vi "Moving Window Waveform Smoother.vi"(9 "Points / Aperture(S)":dbl, 10 "Filter Mode":T1(ring), 11 "Raw Waveforms":waveform(dbl)[](array[waveform])) -> (3 "Filtered Waveforms":waveform(dbl)[](array[waveform]))   [LabVIEW 2010]
uses:
  <vilib>/Analysis/NI_AALBase.lvlib
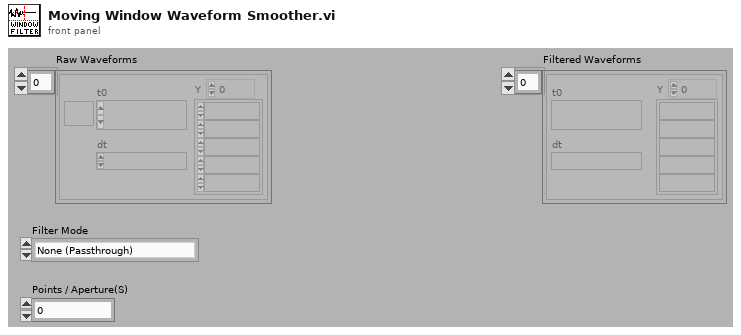
[diagram p1: front panel]
types:
  T1 = enum16{"None (Passthrough)", "Moving Window (Fixed)", "Moving Window (Time)"}
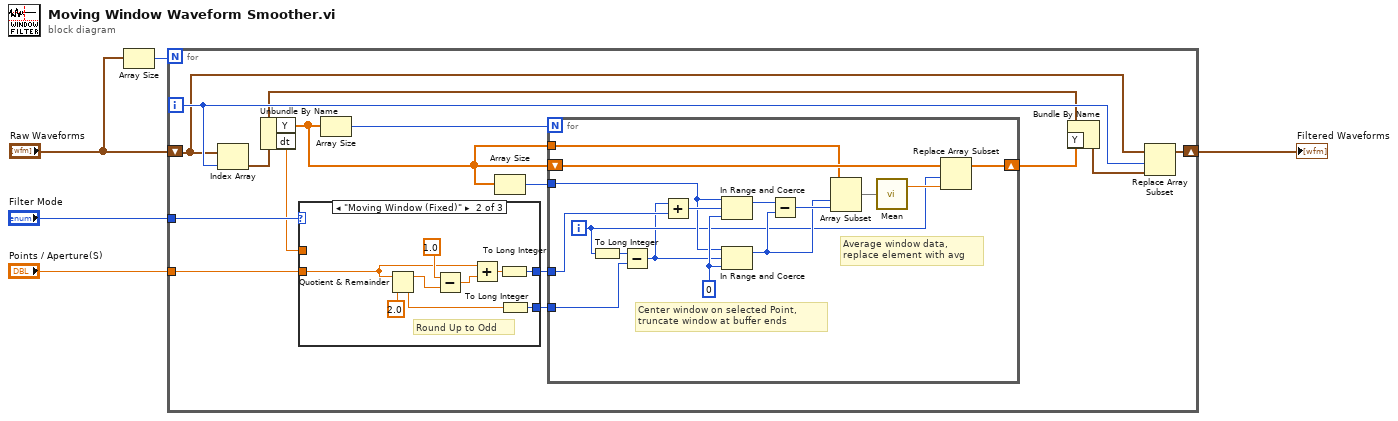
[diagram p0: block diagram]
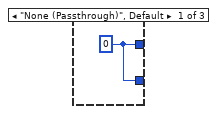
[diagram p2: hidden frame]
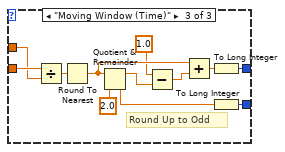
[diagram p3: hidden frame]
diagram:
  n1 = Array Size(array="Raw Waveforms") -> (size(s)=w4:i32)
  n2 = for {
    N: w4 -> [_]
    shift-right: [w9] -> w5
    shift-left: "Raw Waveforms" -> [w18]
    tunnel: "Filter Mode" -> [w13]
    tunnel: "Points / Aperture(S)" -> [w10]
    i -> [w19]
    n3 = Index Array(array=w18, index=w19) -> (element=w16:waveform(dbl))
    n4 = Unbundle By Name(w16) -> ("Y"=w8:dbl[], "dt"=w12:dbl)
    n5 = case shown="\"Moving Window (Fixed)\"" w13 {
      tunnel: w12 -> [_ _ w40]
      tunnel: [w20 w23 w38] -> w11
      tunnel: w10 -> [_ w24 w41]
      tunnel: [w20 w21 w31] -> w6
      frame "None (Passthrough)", Default {
        w20 = 0 ("Points / Aperture(uS)")
      }
      frame "Moving Window (Fixed)" {
        # "Round Up to Odd"
        n6 = Quotient & Remainder(x=w24, y=2.0) -> (x-y*floor(x/y)=w25:dbl, floor(x/y)=w22:dbl)
        n7 = Subtract(x=1.0 ("y"), y=w25) -> (x-y=w27:dbl)
        n8 = Add(x=w24, y=w27) -> (x+y=w28:dbl)
        n9 = To Long Integer(number=w28) -> (32bit integer=w23:i32)
        n10 = To Long Integer(number=w22) -> (32bit integer=w21:i32)
      }
      frame "Moving Window (Time)" {
        # "Round Up to Odd"
        n11 = Divide(x=w41, y=w40) -> (x/y=w39:dbl)
        n12 = Round To Nearest(number=w39) -> (nearest integer value=w36:dbl)
        n13 = Quotient & Remainder(x=w36, y=2.0) -> (x-y*floor(x/y)=w32:dbl, floor(x/y)=w30:dbl)
        n14 = Subtract(x=1.0 ("y"), y=w32) -> (x-y=w34:dbl)
        n15 = Add(x=w36, y=w34) -> (x+y=w35:dbl)
        n16 = To Long Integer(number=w35) -> (32bit integer=w38:i32)
        n17 = To Long Integer(number=w30) -> (32bit integer=w31:i32)
      }
    }
    n18 = Array Size(array=w8) -> (size(s)=w17:i32)
    n19 = Array Size(array=w8) -> (size(s)=w7:i32)
    n20 = for {
      N: w17 -> [_]
      shift-right: [w57] -> w14
      shift-left: w8 -> [w56]
      tunnel: w11 -> [w51]
      tunnel: w8 -> [w55]
      tunnel: w7 -> [w49]
      tunnel: w6 -> [w43]
      i -> [w45]
      w52 = 0 ("lower limit")
      # "Average window data,\nreplace element with avg"
      # "Center window on selected Point,\ntruncate window at buffer ends"
      n21 = To Long Integer(number=w45) -> (32bit integer=w44:i32)
      n22 = Subtract(x=w44, y=w43) -> (x-y=w42:i32)
      n23 = Add(x=w42, y=w51) -> (x+y=w50:i32)
      n24 = In Range and Coerce(upper limit=w49, x=w50, lower limit=w52) -> (coerced(x)=w48:i32)  [unwired: 1 out]
      n25 = In Range and Coerce(upper limit=w49, x=w42, lower limit=w52) -> (coerced(x)=w46:i32)  [unwired: 1 out]
      n26 = Subtract(x=w48, y=w46) -> (x-y=w47:i32)
      n27 = Array Subset(array=w55, index=w46, length=w47) -> (w54:dbl[])
      n28 = call <vilib>:"Mean.vi"("X"=w54) -> ("mean"=w53:dbl)  [unwired: 1 out]
      n29 = Replace Array Subset(array=w56, new element=w53, index=w45) -> (w57:dbl[])
    }
    n30 = Bundle By Name(cluster=w16, "Y"=w14) -> (w15:waveform(dbl))
    n31 = Replace Array Subset(array=w18, new element=w15, index=w19) -> (w9:waveform(dbl)[])
  }
  "Filtered Waveforms" <- w5
